vi "Process OCR.vi"(8 "error in (no error)":errorcluster, 9 "Language":string, 10 "Output File Name":string, 11 "Image Name":string) -> (0 "error out":errorcluster)   [LabVIEW 2019]
uses:
  <vilib>/Utility/file.llb/Write Delimited Spreadsheet (string).vi
panel:
  out "x-y":u32
  out "standard output":string
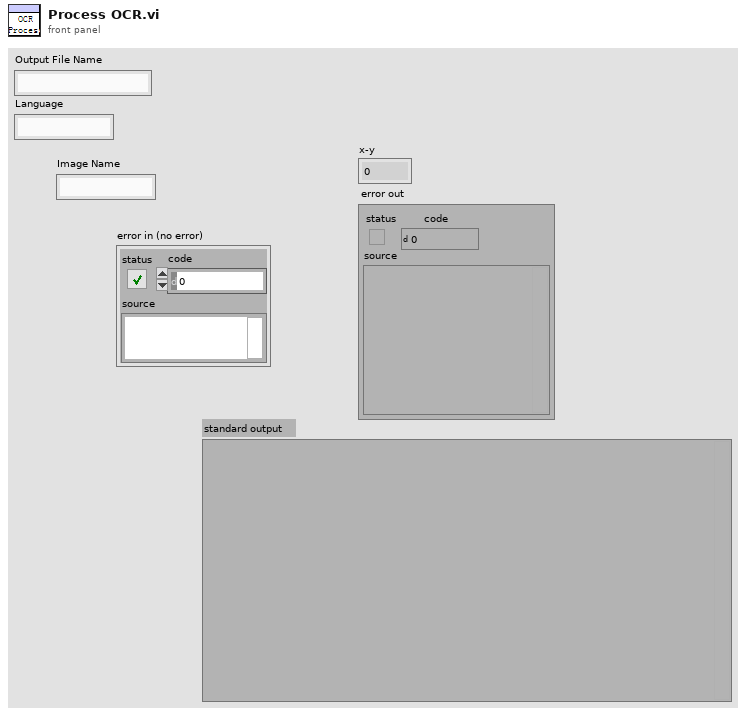
[diagram p1: front panel]
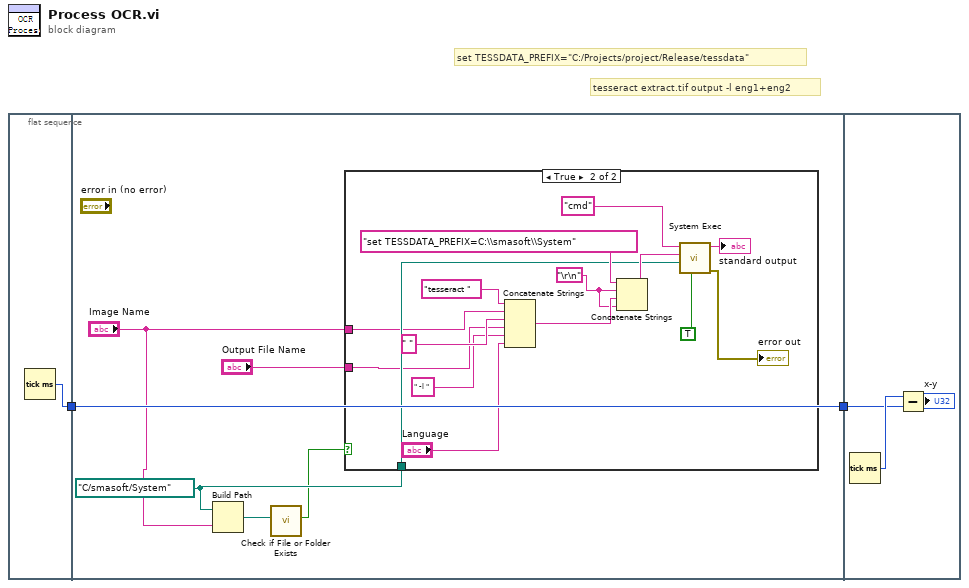
[diagram p0: block diagram]
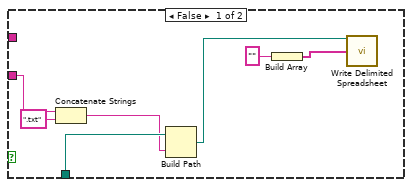
[diagram p2: hidden frame]
diagram:
  # "tesseract extract.tif output -l eng1+eng2"
  # "set TESSDATA_PREFIX=\"C:/Projects/project/Release/tessdata\""
  n1 = flat-sequence {
    tunnel: [w3] -> w1
    tunnel: [w9] -> w2
    tunnel: w1 -> [w9]
    tunnel: w2 -> [w33]
    frame #0 {
      n2 = Tick Count (ms)() -> (millisecond timer value=w3:u32)
    }
    frame #1 {
      w8 = path "C:/smasoft/System" ("working directory")
      n3 = Build Path(base path=w8, name or relative path="Image Name") -> (appended path=w6:path)
      n4 = call <vilib>:"Check if File or Folder Exists.vi"("path"=w6) -> ("file or folder exists?"=w5:bool)  [unwired: 8 in, 2 out]
      n5 = case shown="True" w5 {
        tunnel: w8 -> [w12 w19]
        tunnel: "Image Name" -> [_ w18]
        tunnel: "Output File Name" -> [w14 w17]
        frame False {
          n6 = Concatenate Strings(w14, ".txt" ("string")) -> (w11:string)
          n7 = Build Path(base path=w12, name or relative path=w11) -> (appended path=w10:path)
          n8 = Build Array("") -> (w15:string[])
          n9 = call-poly <vilib>:"Write Delimited Spreadsheet.vi"("file path (dialog if empty)"=w10, "1D data"=w15) -> ()  [unwired: 12 in, 2 out]
        }
        frame True {
          w21 = "\r\n"
          n10 = Concatenate Strings("tesseract " ("command line"), w18, " " ("string"), w17, " -l " ("string"), "Language") -> (w22:string)
          n11 = Concatenate Strings("set TESSDATA_PREFIX=C:\\smasoft\\System" ("standard input"), w21, w22, w21) -> (w20:string)
          n12 = call <vilib>:"System Exec.vi"("run minimized? (F)"=TRUE, "working directory"=w19, "standard input"=w20, "command line"="cmd") -> ("error out"=→"error out":errorcluster, "standard output"=→"standard output":string)  [unwired: 4 in, 2 out]
        }
      }
    }
    frame #2 {
      n13 = Tick Count (ms)() -> (millisecond timer value=w34:u32)
      n14 = Subtract(x=w34, y=w33) -> (x-y=→"x-y":u32)
    }
  }
